vi "ReadCurrent.vi"(8 "error in (no error)":errorcluster, 10 "LoopFromMain":bool, 11 "VISA resource name":refnum<visa-resource-name>="COM9") -> (0 "error out":errorcluster, 2 "CurrentOut":string)   [LabVIEW 2017]
uses:
  <vilib>/Instr/_visa.llb/VISA Configure Serial Port (Instr).vi
panel:
  out "Array":string[](array[string])
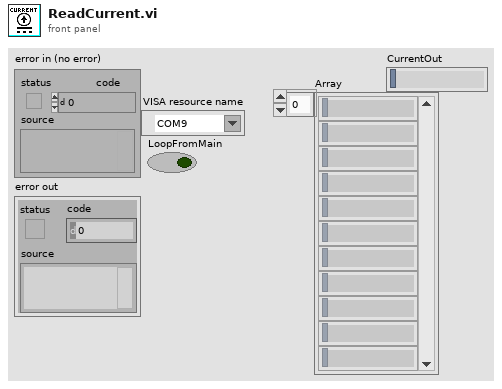
[diagram p1: front panel]
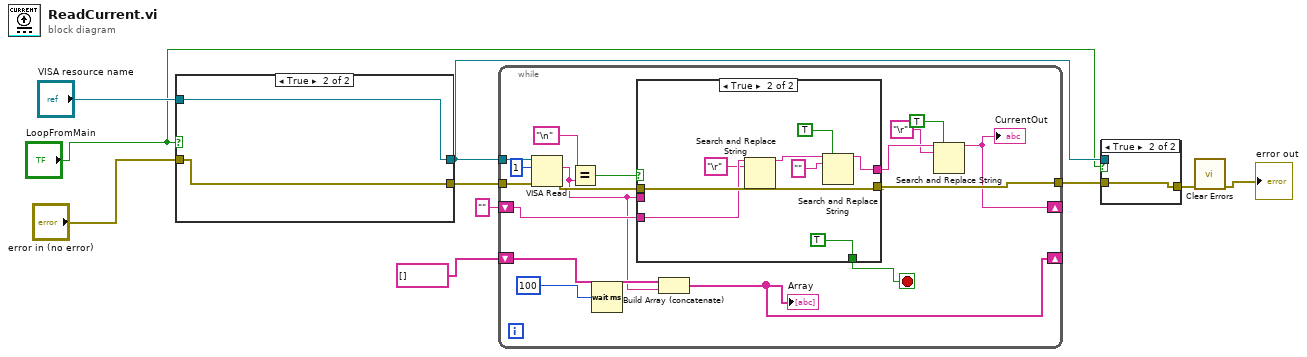
[diagram p0: block diagram]
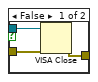
[diagram p2: hidden frame]
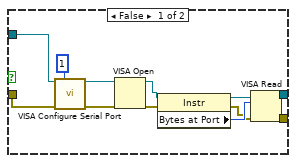
[diagram p3: hidden frame]
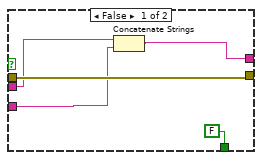
[diagram p4: hidden frame]
diagram:
  n1 = case shown="True" "LoopFromMain" {
    tunnel: [w19 w23] -> w10
    tunnel: "error in (no error)" -> [w16 w23]
    tunnel: "VISA resource name" -> [w14 w24]
    tunnel: [w11 w24] -> w5
    frame False {
      n2 = call-poly "VISA Configure Serial Port"("VISA resource name"=w14, "timeout (10sec)"=u32 1, "error in (no error)"=w16) -> ("VISA resource name out"=w13:refnum<visa-resource-name>, "error out"=w15:errorcluster)  [unwired: 11 in]
      n3 = VISA Open(error in (no error)=w15, VISA resource name=w13) -> (VISA resource name=w22:refnum<visa-resource-name>, error out=w17:errorcluster)  [unwired: 3 in]
      n4 = property class="Instr"(reference=w22, error in=w17) -> (reference out=w20:refnum<visa-resource-name>, error out=w18:errorcluster, "Bytes at Port"=w21:u32)
      n5 = VISA Read(VISA resource name=w20, byte count=w21, error in (no error)=w18) -> (VISA resource name out=w11:refnum<visa-resource-name>, error out=w19:errorcluster)  [unwired: 2 out]
    }
    frame True {
    }
  }
  n6 = while {
    tunnel: w5 -> [w41]
    tunnel: w10 -> [w39]
    tunnel: [w37] -> w4
    shift-right: [w28] -> _
    shift-left: "" -> [w35]
    shift-right: [w29] -> _
    shift-left: string[] [] -> [w31]
    stop <- w34 stop-if-true
    n7 = VISA Read(VISA resource name=w41, byte count=u32 1, error in (no error)=w39) -> (read buffer=w30:string, error out=w38:errorcluster)  [unwired: 2 out]
    n8 = Equal?(x="\n", y=w30) -> (x = y?=w32:bool)
    n9 = Wait (ms)(milliseconds to wait=u32 100) -> ()  [unwired: 1 out]
    n10 = case shown="True" w32 {
      tunnel: [FALSE TRUE] -> w34
      tunnel: w38 -> [w45 w53]
      tunnel: [w45 w53] -> w37
      tunnel: [w42 w47] -> w27
      tunnel: w35 -> [w43 w52]
      tunnel: w30 -> [w44 _]
      frame False {
        n11 = Concatenate Strings(w44, w43) -> (w42:string)
      }
      frame True {
        n12 = Search and Replace String(input string=w52, search string="\r") -> (result string=w50:string)  [unwired: 6 in, 3 out]
        n13 = Search and Replace String(replace all?=TRUE ("replace all? (F)"), input string=w50, search string="") -> (result string=w47:string)  [unwired: 5 in, 3 out]
      }
    }
    n14 = Build Array (concatenate)(w31, w30) -> (w29:string[])
    "Array" <- w29
    n15 = Search and Replace String(replace all?=TRUE ("replace all? (F)"), input string=w27, search string="\r") -> (result string=w28:string)  [unwired: 5 in, 3 out]
    "CurrentOut" <- w28
  }
  n16 = case shown="True" "LoopFromMain" {
    tunnel: w5 -> [w57 _]
    tunnel: w4 -> [w56 w58]
    tunnel: [w55 w58] -> w3
    frame False {
      n17 = VISA Close(VISA resource name=w57, error in (no error)=w56) -> (error out=w55:errorcluster)
    }
    frame True {
    }
  }
  n18 = call <vilib>:"Clear Errors.vi"("error in (no error)"=w3) -> ("error out"=→"error out":errorcluster)  [unwired: 5 in, 1 out]
